vi "FlatToRichstreamai_waveform.vi"(5 "OutputClusterType":T1, 11 "InputCluster":T3) -> (3 "OutputCluster":T1)   [LabVIEW 2023, in "Generated_server.lvlib"]
uses:
  Generated_server.lvlib
  streamai_waveform_Flat.ctl
  google_protobuf_Timestamp_Flat.ctl
  streamai_waveform.ctl
  google_protobuf_Timestamp.ctl
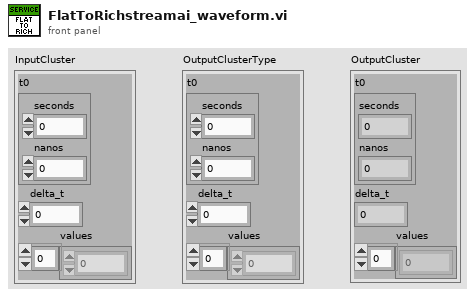
[diagram p1: front panel]
types:
  T1 = typedef "Generated_server.lvlib/streamai_waveform.ctl" = cluster{"t0":T2, "delta_t":dbl, "values":dbl[]}
  T2 = typedef "Generated_server.lvlib/google_protobuf_Timestamp.ctl" = cluster{"seconds":i64, "nanos":i32}
  T3 = typedef "Generated_server.lvlib/streamai_waveform_Flat.ctl" = cluster{"t0":T4, "delta_t":dbl, "values":dbl[]}
  T4 = typedef "Generated_server.lvlib/google_protobuf_Timestamp_Flat.ctl" = cluster{"seconds":i64, "nanos":i32}
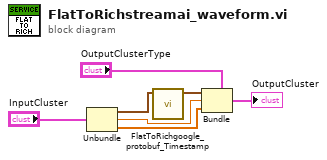
[diagram p0: block diagram]
diagram:
  n1 = Unbundle "Unbundle"("InputCluster") -> ("t0"=w4:T4, "delta_t"=w2:dbl, "values"=w1:dbl[])
  n2 = call "FlatToRichgoogle_protobuf_Timestamp.vi"("InputCluster"=w4) -> ("OutputCluster"=w3:T2)  [unwired: 10 in]
  n3 = Bundle "Bundle"(cluster="OutputClusterType", "t0"=w3, "delta_t"=w2, "values"=w1) -> (→"OutputCluster":T1)
